vi "Eat.vi"(8 "error in (no error)":errorcluster, 10 "SnakeGame in":refnum<class "SnakeGame.lvclass">, 11 "Snake in":refnum<class "Snake.lvclass">) -> (0 "error out":errorcluster, 2 "SnakeGame out":refnum<class "SnakeGame.lvclass">, 3 "Snake out":refnum<class "Snake.lvclass">)   [LabVIEW 2019, in "RT_Game.lvlib" / "Snake.lvclass"]
uses:
  Snake.lvclass
  SnakeGame/SnakeGame.lvclass
  Snake.lvclass/Snake.ctl
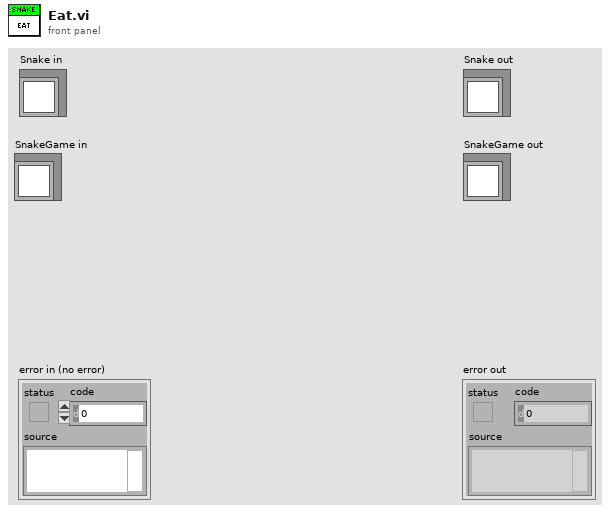
[diagram p1: front panel]
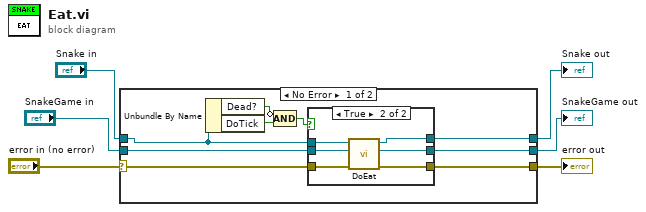
[diagram p0: block diagram]
diagram:
  n1 = case shown="No Error" "error in (no error)" {
    selector: "error in (no error)" -> [w15 w27]
    tunnel: [w14 w27] -> w5
    tunnel: [w11 w26] -> w3
    tunnel: "Snake in" -> [w10 w26]
    tunnel: [w13 w25] -> w2
    tunnel: "SnakeGame in" -> [w12 w25]
    frame No Error {
      n2 = Unbundle By Name(w10) -> ("Dead?"=w9:bool, "DoTick"=w8:bool)
      n3 = Compound Arithmetic op=AND(invert w9, w8) -> (w7:bool)
      n4 = case shown="True" w7 {
        tunnel: w15 -> [w16 w24]
        tunnel: [w16 w23] -> w14
        tunnel: [w17 w22] -> w13
        tunnel: w12 -> [w17 w21]
        tunnel: w10 -> [w18 w20]
        tunnel: [w18 w19] -> w11
        frame False {
        }
        frame True {
          n5 = call "DoEat.vi"("error in (no error)"=w24, "SnakeGame in"=w21, "Snake in"=w20) -> ("error out"=w23:errorcluster, "SnakeGame out"=w22:refnum<class "SnakeGame.lvclass">, "Snake out"=w19:refnum<class "Snake.lvclass">)  [unwired: 6 in]
        }
      }
    }
    frame Error {
    }
  }
  "error out" <- w5
  "Snake out" <- w3
  "SnakeGame out" <- w2
